vi "スプリッタ 1.vi"() -> ()   [LabVIEW 2016]
panel:
  in  "サブパネル選択":i16
  in  "環境設定ボタン":bool
  in  "再生設定ボタン":bool
  in  "終了ボタン":bool
  in  "再生ボタン":bool
  in  "記録ボタン":bool
  in  "記録設定ボタン":bool
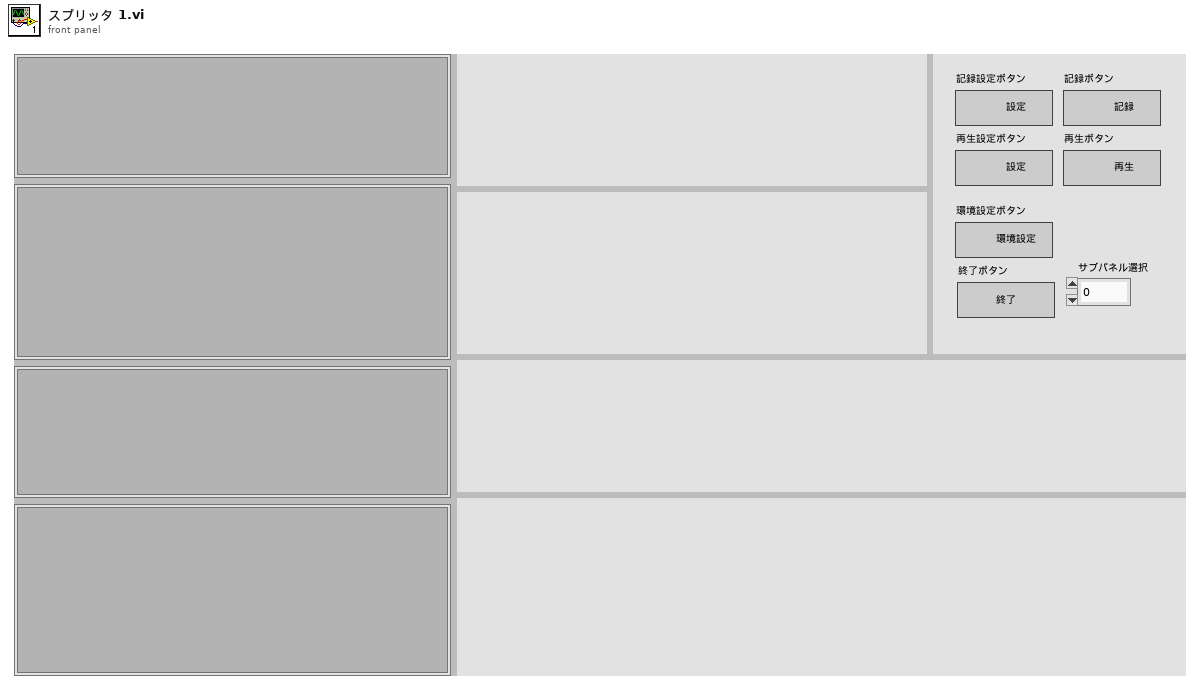
[diagram p1: front panel]
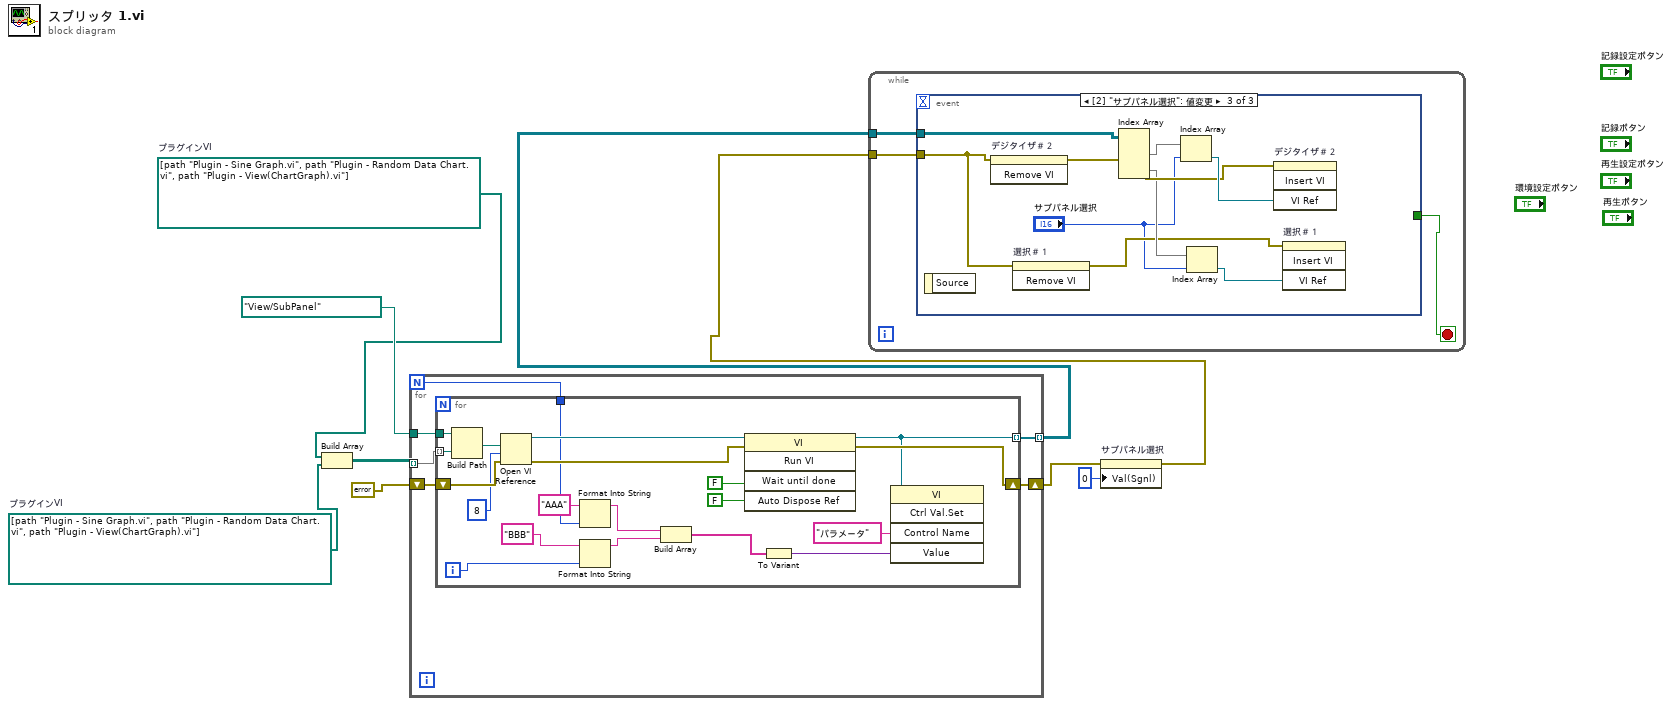
[diagram p0: block diagram]
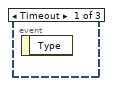
[diagram p2: hidden frame]
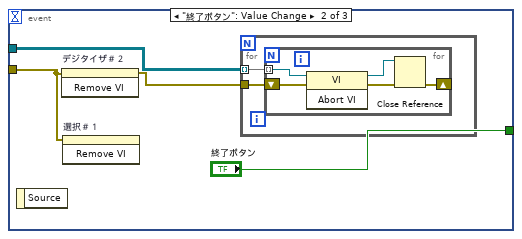
[diagram p3: hidden frame]
diagram:
  w2 = path[] [path "Plugin - Sine Graph.vi", path "Plugin - Random Data Chart.vi", path "Plugin - View(ChartGraph).vi"]  # プラグインVI
  w3 = path[] [path "Plugin - Sine Graph.vi", path "Plugin - Random Data Chart.vi", path "Plugin - View(ChartGraph).vi"]  # プラグインVI
  n1 = Build Array(w3, w2) -> (w1:path[][])
  n2 = for {
    N -> [w10]
    tunnel: w1 -> [w14] mode=indexing
    tunnel: path "View/SubPanel" -> [w15]
    shift-right: [w12] -> w7
    shift-left: errorcluster {"status"=FALSE, "code"=0, "source"=""} ("error constant") -> [w13]
    tunnel: [w11] -> w5 mode=indexing
    n3 = for {
      tunnel: w15 -> [w35]
      tunnel: w14 -> [w34] mode=indexing
      tunnel: [w25] -> w11 mode=indexing
      shift-right: [w27] -> w12
      shift-left: w13 -> [w28]
      tunnel: w10 -> [w23]
      i -> [w21]
      n4 = Build Path(base path=w35, name or relative path=w34) -> (appended path=w33:path)
      n5 = Open VI Reference(vi path=w33, options=8 ("オプション"), error in (no error)=w28) -> (vi reference=w32:refnum<vi>, error out=w31:errorcluster)  [unwired: 3 in]
      n6 = Format Into String(initial string="AAA" ("初期文字列"), w23) -> (resulting string=w19:string)  [unwired: 2 in, 1 out]
      n7 = Format Into String(initial string="BBB" ("初期文字列"), w21) -> (resulting string=w18:string)  [unwired: 2 in, 1 out]
      n8 = Build Array(w19, w18) -> (w17:string[])
      n9 = invoke on="Invoke Node" class="VI" method="Run VI"(reference=w32, error in=w31, "Wait until done"=FALSE ("Wait Until Done"), "Auto Dispose Ref"=FALSE ("Auto Dispose Reference")) -> (reference out=w25:refnum<vi>, error out=w27:errorcluster)  [unwired: 1 in, 3 out]
      n10 = To Variant(anything=w17) -> (Variant=w16:variant)
      n11 = invoke class="VI" method="Ctrl Val.Set"(reference=w25, "Control Name"="パラメータ" ("制御器名"), "Value"=w16) -> ()  [unwired: 2 in, 5 out]
    }
  }
  n12 = property on="サブパネル選択" class="DigNum （指定）"(error in=w7, "Val(Sgnl)"=i16 0 ("値（信号）")) -> (error out=w4:errorcluster)  [unwired: 1 in, 1 out]
  n13 = while {
    tunnel: w5 -> [w37]
    tunnel: w4 -> [w36]
    stop <- w38 stop-if-true
    n14 = event shown="[2] \"サブパネル選択\": 値変更" {
      selector: _ -> [_ _ _]
      dyn-events: _ -> [_ _ _]
      timeout: _ -> [_ _ _]
      tunnel: [_ "終了ボタン" _] -> w38
      tunnel: w37 -> [_ w41 w55]
      tunnel: w36 -> [_ w39 w56]
      event Timeout {
        n15 = event-data() -> ()  [unwired: 1 in, 1 out]
      }
      event "終了ボタン": Value Change {
        n16 = event-data() -> ()  [unwired: 1 in, 1 out]
        n17 = invoke on="デジタイザ＃２" class="SubPnl" method="Remove VI"(error in=w39) -> (error out=w40:errorcluster)  [unwired: 2 in, 2 out]
        n18 = invoke on="選択＃１" class="SubPnl" method="Remove VI"(error in=w39) -> ()  [unwired: 2 in, 3 out]
        n19 = for {
          tunnel: w41 -> [w44] mode=indexing
          tunnel: w40 -> [w43]
          n20 = for {
            shift-right: [w45] -> _
            shift-left: w43 -> [w49]
            tunnel: w44 -> [w48] mode=indexing
            n21 = invoke on="Invoke Node" class="VI" method="Abort VI"(reference=w48, error in=w49) -> (reference out=w46:refnum<vi>, error out=w47:errorcluster)  [unwired: 1 in, 1 out]
            n22 = Close Reference(reference=w46, error in (no error)=w47) -> (error out=w45:errorcluster)
          }
        }
      }
      event "サブパネル選択": Value Change {
        n23 = event-data() -> ()  [unwired: 1 in, 1 out]
        n24 = invoke on="デジタイザ＃２" class="SubPnl" method="Remove VI"(error in=w56) -> (error out=w57:errorcluster)  [unwired: 2 in, 2 out]
        n25 = invoke on="選択＃１" class="SubPnl" method="Remove VI"(error in=w56) -> (error out=w51:errorcluster)  [unwired: 2 in, 2 out]
        n26 = Index Array(array=w55) -> (element #1=w54:refnum<vi>[], element #2=w53:refnum<vi>[])  [unwired: 4 in]
        n27 = Index Array(array=w54, index="サブパネル選択") -> (element=w58:refnum<vi>)
        n28 = Index Array(array=w53, index="サブパネル選択") -> (element=w52:refnum<vi>)
        n29 = invoke on="デジタイザ＃２" class="SubPnl" method="Insert VI"(error in=w57, "VI Ref"=w58) -> ()  [unwired: 2 in, 4 out]
        n30 = invoke on="選択＃１" class="SubPnl" method="Insert VI"(error in=w51, "VI Ref"=w52) -> ()  [unwired: 2 in, 4 out]
      }
    }
  }
